vi "Open FITS [I16-I32-SGL].vi"(0 "Input File:":path) -> (1 "File Read:":path, 6 "Image":sgl[][](array[numeric]) format="%.4f", 14 "Message":string)   [LabVIEW 2022 SP3]
doc: "This VI creates a new datalog file and writes the specified number of records to the file. Each record is a cluster containing a string and an array of single precision numbers."
uses:
  <vilib>/Analysis/NI_AALBase.lvlib
panel:
  out "Header":string
  out "Data Type":string
  out "error out":errorcluster
  in  "AutoscaleON/OFF":bool
  out "RMS":dbl=0.8932524839036273 format="%.2f"
  out "Image":sgl[][](graph)
  out "Mean":dbl=-0.11 format="%.2f"
  out "Slice":sgl[][](graph)
  in  "Box Size":i32=10
  out "Filesize":i32=146880
  out "Image Offset":i32=145476
  # "Macintosh HD:BAM DATA:2004_data:20040427:AlPlate:H_10sec.F16.004.fits"
  # "Macintosh HD:BAM DATA:2004_data:20040425:H_10sec.005.fits"
  # "`"
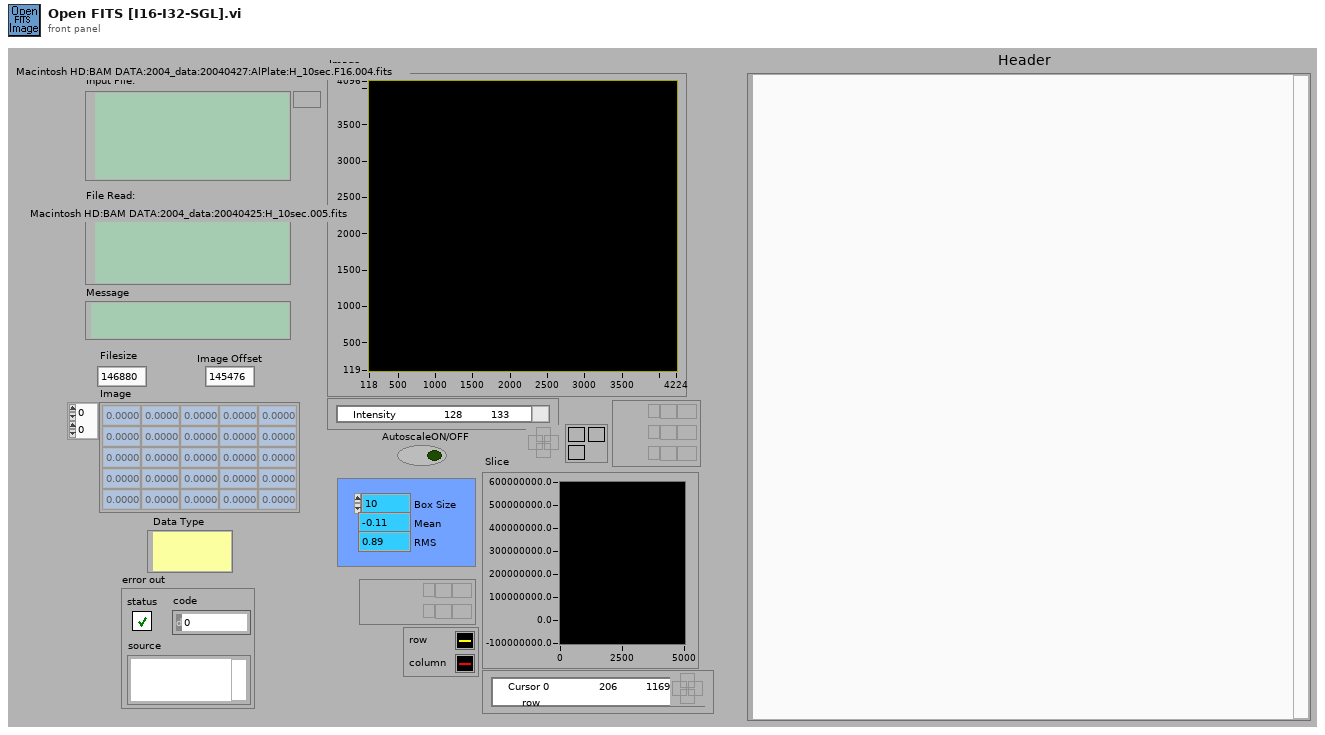
[diagram p1: front panel]
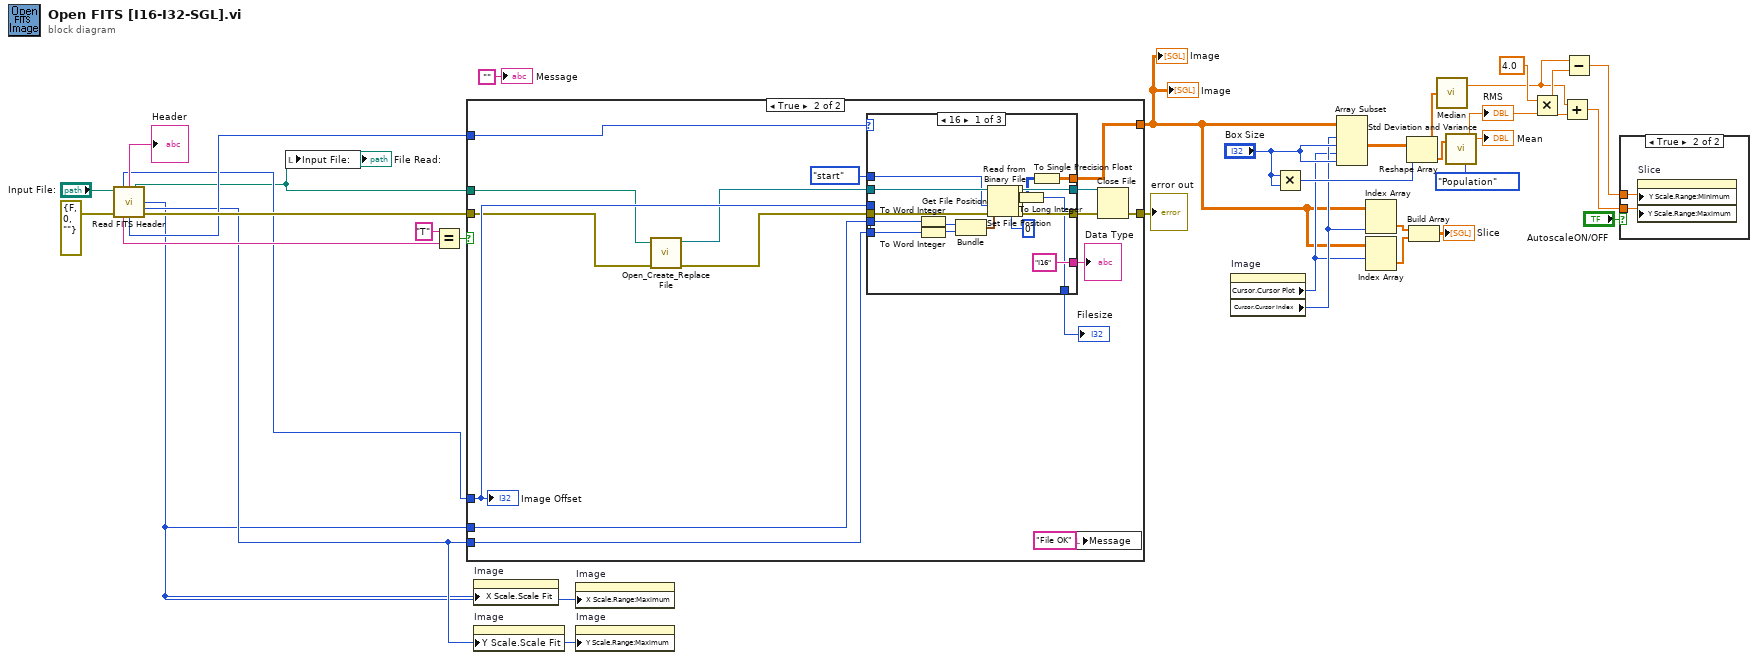
[diagram p0: block diagram]
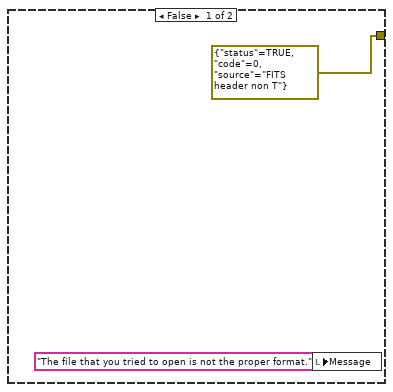
[diagram p2: hidden frame]
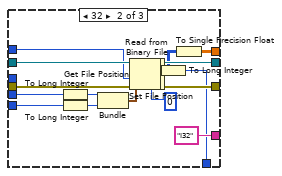
[diagram p3: hidden frame]
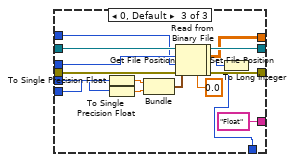
[diagram p4: hidden frame]
diagram:
  n1 = call "Read FITS Header.vi"("Input File:"="Input File:", "error in"=errorcluster {"status"=FALSE, "code"=0, "source"=""} ("error in (no error)")) -> ("Header length"=w2:i32, "Header"=→"Header":string, "File Read:"=w1:path, "NAXIS1"=w6:i32, "NAXIS2"=w7:i32, "SIMPLE"=w9:string, "BITPIX"=w8:i32, "error out"=w12:errorcluster)  [unwired: 4 in, 2 out]
  "File Read:" <- w1
  n2 = local write "Input File:"(w1) -> ()
  n3 = Equal?(x="T", y=w9) -> (x = y?=w14:bool)
  n4 = case shown="True" w14 {
    tunnel: [errorcluster {"status"=TRUE, "code"=0, "source"="FITS header non T"} ("error out") w51] -> w15
    tunnel: w12 -> [_ w41]
    tunnel: w2 -> [_ w47]
    tunnel: [_ w48] -> w10
    tunnel: w7 -> [_ w45]
    tunnel: w6 -> [_ w44]
    tunnel: w8 -> [_ w36]
    tunnel: w1 -> [_ w38]
    frame False {
      n5 = local write "Message"("The file that you tried to open is not the proper format.") -> ()
    }
    frame True {
      n6 = call <vilib>:"Open_Create_Replace File.vi"("error in (no error)"=w41, "file path"=w38) -> ("error out"=w40:errorcluster, "refnum"=w39:refnum<file>)  [unwired: 6 in, 2 out]
      n7 = case shown="16" w36 {
        tunnel: w39 -> [w69 w89 w111]
        tunnel: [w68 w88 w110] -> w50
        tunnel: w40 -> [w67 w87 w108]
        tunnel: [w66 w86 w109] -> w49
        tunnel: w47 -> [_ _ w107]
        tunnel: [w60 w81 w106] -> w48
        tunnel: w45 -> [w64 w84 w99]
        tunnel: w44 -> [w63 w85 w98]
        tunnel: enum16{"start", "end", "current"}."start" ("pos mode (0:2)") -> [w59 w80 w101]
        tunnel: ["I16" "I32" "Float"] -> w42
        tunnel: [w57 w77 w97] -> w37
        frame 16 {
          n8 = To Word Integer(number=w64) -> (16bit integer=w71:i16)
          n9 = To Word Integer(number=w63) -> (16bit integer=w70:i16)
          n10 = Bundle(w71, w70) -> (w62:cluster{i16, i16})  [unwired: 1 in]
          n11 = Set File Position(refnum=w69, from (0:start)=w59, error in=w67) -> (refnum out=w56:refnum<file>, error out=w55:errorcluster)  [unwired: 1 in]
          n12 = Read from Binary File(5:i16 0, 8:w55, 10:w62, 11:w56) -> (0:w53:errorcluster, 2:w65:i16[][], 3:w54:refnum<file>)  [unwired: 2 in, 1 out]
          n13 = Get File Position(4:w53, 7:w54) -> (0:w66:errorcluster, 2:w52:i64, 3:w68:refnum<file>)
          n14 = To Long Integer(number=w52) -> (32bit integer=w57:i32)
          n15 = To Single Precision Float(number=w65) -> (single precision float=w60:sgl[][])
        }
        frame 32 {
          n16 = To Long Integer(number=w85) -> (32bit integer=w91:i32)
          n17 = To Long Integer(number=w84) -> (32bit integer=w90:i32)
          n18 = Bundle(w91, w90) -> (w83:cluster{i32, i32})  [unwired: 1 in]
          n19 = Set File Position(refnum=w89, from (0:start)=w80, error in=w87) -> (refnum out=w76:refnum<file>, error out=w75:errorcluster)  [unwired: 1 in]
          n20 = Read from Binary File(5:0 ("BitPix"), 8:w75, 10:w83, 11:w76) -> (0:w73:errorcluster, 2:w82:i32[][], 3:w74:refnum<file>)  [unwired: 2 in, 1 out]
          n21 = Get File Position(4:w73, 7:w74) -> (0:w86:errorcluster, 2:w72:i64, 3:w88:refnum<file>)
          n22 = To Long Integer(number=w72) -> (32bit integer=w77:i32)
          n23 = To Single Precision Float(number=w82) -> (single precision float=w81:sgl[][])
        }
        frame 0, Default {
          n24 = To Single Precision Float(number=w99) -> (single precision float=w104:sgl)
          n25 = To Single Precision Float(number=w98) -> (single precision float=w105:sgl)
          n26 = Bundle(w104, w105) -> (w103:cluster{sgl, sgl})  [unwired: 1 in]
          n27 = Set File Position(offset (in bytes) (0)=w107, refnum=w111, from (0:start)=w101, error in=w108) -> (refnum out=w96:refnum<file>, error out=w95:errorcluster)
          n28 = Read from Binary File(5:sgl 0.0, 8:w95, 10:w103, 11:w96) -> (0:w93:errorcluster, 2:w106:sgl[][], 3:w94:refnum<file>)  [unwired: 2 in, 1 out]
          n29 = Get File Position(4:w93, 7:w94) -> (0:w109:errorcluster, 2:w92:i64, 3:w110:refnum<file>)
          n30 = To Long Integer(number=w92) -> (32bit integer=w97:i32)
        }
      }
      "Data Type" <- w42
      "Filesize" <- w37
      n31 = local write "Message"("File OK") -> ()
      n32 = Close File(refnum=w50, error in=w49) -> (error out=w51:errorcluster)  [unwired: 1 out]
      "Image Offset" <- w47
    }
  }
  "error out" <- w15
  "Image" <- w10
  "Image" <- w10
  n33 = property on="Image" class="IntGraph (strict)"("X Scale.Scale Fit"=w6) -> ()  [unwired: 2 in, 2 out]
  n34 = property on="Image" class="IntensityGraph (strict)"("Y Scale.Scale Fit"=w7) -> ()  [unwired: 2 in, 2 out]
  n35 = property on="Image" class="IntGraph (strict)"("X Scale.Range:Maximum"=w6) -> ()  [unwired: 2 in, 2 out]
  n36 = property on="Image" class="IntGraph (strict)"("Y Scale.Range:Maximum"=w7) -> ()  [unwired: 2 in, 2 out]
  n37 = property on="Image" class="IntGraph (strict)"() -> ("Cursor.Cursor Plot"=w11:i32, "Cursor.Cursor Index"=w17:i32)  [unwired: 2 in, 2 out]
  n38 = Multiply(x="Box Size", y="Box Size") -> (x*y=w33:i32)
  n39 = Array Subset(array=w10, index (row)=w17, length (row)="Box Size", index (col)=w11, length (col)="Box Size") -> (w29:sgl[][])
  n40 = Index Array(array=w10, index (col)=w17) -> (element=w31:sgl[])  [unwired: 1 in]
  n41 = Index Array(array=w10, index (row)=w11) -> (element=w30:sgl[])  [unwired: 1 in]
  n42 = Reshape Array(w29, w33) -> (w32:sgl[])
  n43 = Build Array(w31, w30) -> (→"Slice":sgl[][])
  n44 = call <vilib>:"Median.vi"("X"=w32) -> ("median"=w23:dbl)  [unwired: 1 out]
  n45 = call <vilib>:"Std Deviation and Variance.vi"("X"=w32, "Weighting (Sample)"=enum16{"Sample", "Population"}."Population") -> ("mean"=→"Mean":dbl, "standard deviation"=w28:dbl)  [unwired: 1 out]
  "RMS" <- w28
  n46 = Multiply(x=4.0, y=w28) -> (x*y=w24:dbl)
  n47 = Add(x=w23, y=w24) -> (x+y=w21:dbl)
  n48 = Subtract(x=w23, y=w24) -> (x-y=w22:dbl)
  n49 = case shown="True" "AutoscaleON/OFF" {
    tunnel: w22 -> [_ w113]
    tunnel: w21 -> [_ w112]
    frame False {
    }
    frame True {
      n50 = property on="Slice" class="WFGraph (strict)"("Y Scale.Range:Minimum"=w113, "Y Scale.Range:Maximum"=w112) -> ()  [unwired: 2 in, 2 out]
    }
  }
  "Message" <- ""
